vi "lp-server.vi"() -> ()   [LabVIEW 2014]
uses:
  lvnanomsg/nanomsg_context.lvclass
  lvnanomsg/nanomsg_socket.lvclass
  lvnanomsg/nanomsg.lvlib
panel:
  in  "stop?":bool
  out "loop":i32
  in  "endpoint":string="tcp://127.0.0.1:5555"
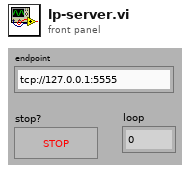
[diagram p1: front panel]
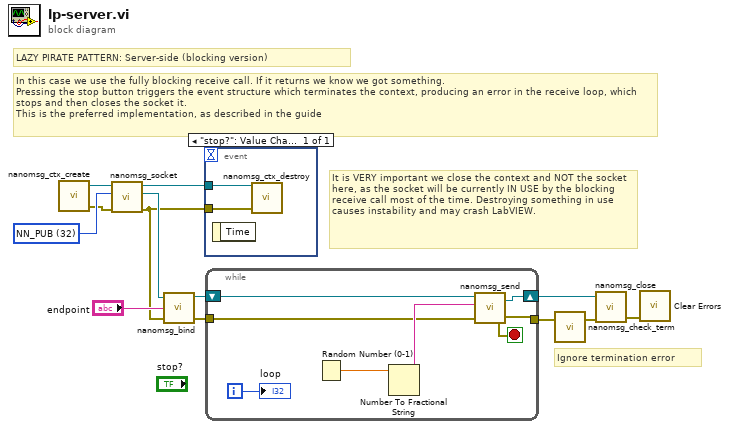
[diagram p0: block diagram]
diagram:
  w4 = 32 items=["NN_WS"=-4, "NN_TCP"=-3, "NN_IPC"=-2, "NN_INPROC"=-1, "NN_SOL_SOCKET"=0, "NN_PAIR"=16, "NN_PUB"=32, "NN_SUB"=33, "NN_REQ"=48, "NN_REP"=49, "NN_PUSH"=80, "NN_PULL"=81, "NN_SURVEYOR"=98, "NN_RESPONDENT"=99, "NN_BUS"=112] ("socket levels")
  # "Ignore termination error"
  # "It is VERY important we close the context and NOT the socket here, as the socket will be currently IN USE by the blocking receive call most of the time. Destroying something in use causes instability and may crash LabVIEW."
  # "In this case we use the fully blocking receive call. If it returns we know we got something.\nPressing the stop button triggers the event structure which terminates the context, producing an error in the receive loop, which stops and then closes the socket it.\nThis is the preferred implementation, as described in the guide"
  # "LAZY PIRATE PATTERN: Server-side (blocking version)"
  n1 = call "nanomsg_ctx_create.vi"() -> ("error out"=w1:errorcluster, "context out"=w10:refnum<class "nanomsg_context.lvclass">)  [unwired: 4 in]
  n2 = call "nanomsg_socket.vi"("error in"=w1, "socket type"=w4, "context in"=w10) -> ("error out"=w3:errorcluster, "socket out"=w9:refnum<class "nanomsg_socket.lvclass">, "context out"=w8:refnum<class "nanomsg_context.lvclass">)  [unwired: 2 in]
  n3 = call "nanomsg_bind.vi"("error in"=w3, "endpoint"="endpoint", "socket in"=w9) -> ("error out"=w2:errorcluster, "socket out"=w12:refnum<class "nanomsg_socket.lvclass">)  [unwired: 1 in]
  n4 = event shown="[0] \"stop?\": Value Change" {
    selector: _ -> [_]
    dyn-events: _ -> [_]
    timeout: _ -> [_]
    tunnel: w8 -> [w15]
    tunnel: w3 -> [w14]
    event "stop?": Value Change {
      n5 = event-data() -> ()  [unwired: 1 in, 1 out]
      n6 = call "nanomsg_ctx_destroy.vi"("error in"=w14, "context in"=w15) -> ()  [unwired: 3 in, 1 out]
    }
  }
  n7 = while {
    shift-right: [w22] -> w11
    shift-left: w12 -> [w18]
    tunnel: [w20] -> w6
    tunnel: w2 -> [w17]
    i -> [w21]
    stop <- w20 stop-if-true
    n8 = Random Number (0-1)() -> (number: 0 to 1=w16:dbl)
    n9 = Number To Fractional String(number=w16) -> (F-format string=w19:string)  [unwired: 3 in]
    n10 = call "nanomsg_send.vi"("error in"=w17, "data"=w19, "socket in"=w18) -> ("error out"=w20:errorcluster, "socket out"=w22:refnum<class "nanomsg_socket.lvclass">)  [unwired: 1 in]
    "loop" <- w21
  }
  n11 = call "nanomsg_check_term.vi"("error in"=w6) -> ("error out"=w5:errorcluster)  [unwired: 1 in, 1 out]
  n12 = call "nanomsg_close.vi"("error in"=w5, "socket"=w11) -> ("error out"=w7:errorcluster)  [unwired: 3 in]
  n13 = call <vilib>:"Clear Errors.vi"("error in (no error)"=w7) -> ()  [unwired: 5 in, 2 out]
